vi "ConnectRobot.vi"(0 "Universal Robot.lvclass in":refnum<class "Universal Robot.lvclass">, 5 "error in (no error)":errorcluster) -> (14 "Universal Robot.lvclass out":refnum<class "Universal Robot.lvclass">, 19 "error out":errorcluster)   [LabVIEW 2019, in "Universal Robot.lvclass"]
uses:
  Universal Robot.lvclass
  Universal Robot.lvclass/Universal Robot.ctl
  Client Interfaces/Dashboard Server/Dashboard Server.lvclass
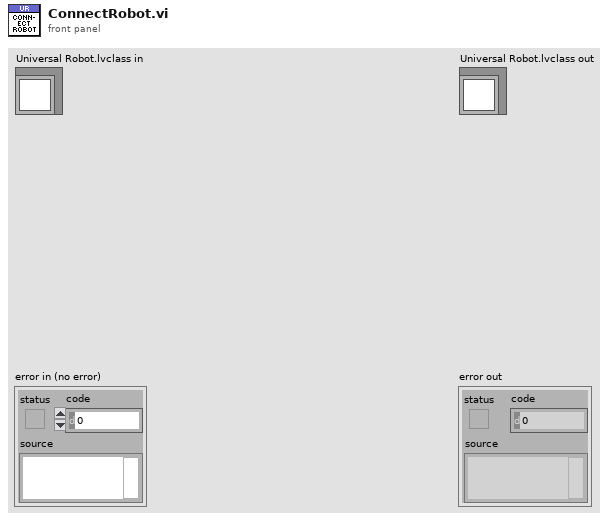
[diagram p1: front panel]
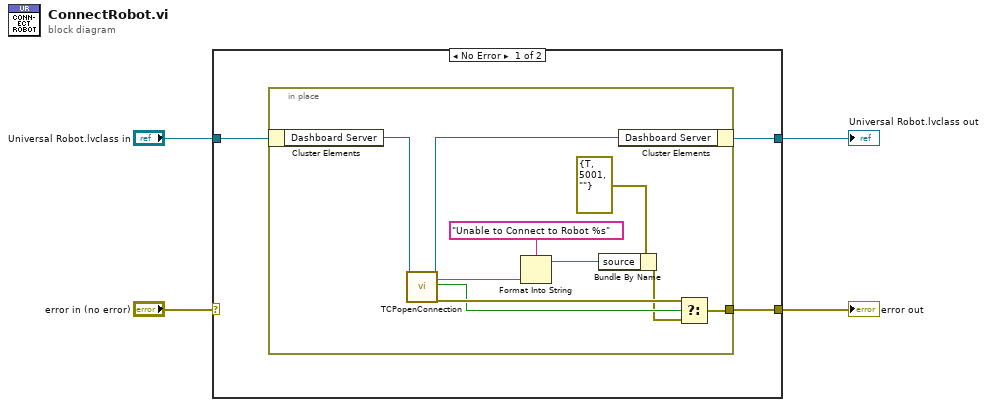
[diagram p0: block diagram]
diagram:
  n1 = case shown="No Error" "error in (no error)" {
    selector: "error in (no error)" -> [_ w19]
    tunnel: [w7 w19] -> w3
    tunnel: "Universal Robot.lvclass in" -> [w6 w18]
    tunnel: [w5 w18] -> w1
    frame No Error {
      n2 = in-place {
        in-place-border: [w11] -> w7
        n3 = in-place-cluster #1(w6) -> ("Dashboard Server"=w9:refnum<class "Dashboard Server.lvclass">)
        n4 = call-dynamic "TCPopenConnection.vi"("DashboardServer in"=w9) -> ("DashboardServer out"=w8:refnum<class "Dashboard Server.lvclass">, "connectionStatus"=w15:string, "connected"=w16:bool, "error out"=w17:errorcluster)  [unwired: 15 in]
        n5 = Format Into String(format string="Unable to Connect to Robot %s", w15) -> (resulting string=w13:string)  [unwired: 2 in, 1 out]
        n6 = Bundle By Name(cluster=errorcluster {"status"=TRUE, "code"=5001, "source"=""} ("error constant"), "source"=w13) -> (w12:errorcluster)
        n7 = in-place-cluster #1("Dashboard Server"=w8) -> (w5:refnum<class "Universal Robot.lvclass">)
        n8 = Select(t=w17, s=w16, f=w12) -> (s? t:f=w11:errorcluster)
      }
    }
    frame Error {
    }
  }
  "error out" <- w3
  "Universal Robot.lvclass out" <- w1
